vi "Double FFT Mesurament (Max Bin detection - Control - Init Wave&Window - Snapshot - DoubleFFT - Latency) RT Test.vi"() -> ()   [LabVIEW 2014]
uses:
  <vilib>/Platform/TimedLoop/XDataNode/timing_clust.ctl
  <vilib>/Platform/TimedLoop/XDataNode/nitl_modes.ctl
  <vilib>/Platform/TimedLoop/XDataNode/wakeup.ctl
  <vilib>/FPGAPlugInAG/sbRIO-9636/niLvFpga_Open_sbRIO-9636.vi
  <vilib>/rvi/interface/common/dynamic/niFpgaDynamicAddResources.vi
  <vilib>/Utility/error.llb/Error Cluster From Error Code.vi
  <vilib>/rvi/errors/niLvFpgaAdjustHostInterfaceError.vi
  <vilib>/rvi/interface/common/niFpgaWaitOnOcc.vi
  <vilib>/FPGAPlugInAG/Dynamic/niLvFpga_Run_Dynamic.vi
  <vilib>/FPGAPlugInAG/Dynamic/niLvFpga_Abort_Dynamic.vi
  <vilib>/FPGAPlugInAG/Dynamic/niLvFpga_Reset_Dynamic.vi
  <vilib>/FPGAPlugInAG/Dynamic/niLvFpga_Close_Dynamic.vi
  <vilib>/rvi/interface/nirviOpenFPGA/nirviOpenFPGA.xnode
  FPGA Bitfiles/LaserDistanceSen_FPGATarget_DoubleFFTMesuram_3rzWOSKuVyU.lvbitx
  FPGA Target/Test VIs/Double FFT Mesurament (Max Bin detection - Control - Init Wave&Window - Snapshot - DoubleFFT - Latency) test.vi
  <vilib>/rvi/interface/nirviReadWriteControl/nirviReadWriteControl.xnode
  <vilib>/rvi/interface/nirviMethod/nirviMethod.xnode
  <vilib>/Platform/TimedLoop/XDataNode/XDataNode.xnode
  <vilib>/rvi/interface/nirviCloseFPGA/nirviCloseFPGA.xnode
  <vilib>/FPGAPlugInAG/Dynamic/niLvFpga_ConfigureFifo_Dynamic.vi
  <vilib>/rvi/errors/niLvFpgaMergeErrorWithErrorCode.vi
  <vilib>/FPGAPlugInAG/Dynamic/niLvFpga_StartFifo_Dynamic.vi
  <vilib>/rvi/interface/Simulation/niFpgaSimulationCallBeginRW.vi
  <vilib>/FPGAPlugInAG/Dynamic/niLvFpga_ReadFifo_Dynamic.vi
  <vilib>/Platform/TimedLoop/XDataNode/XDNodeRunTimeDep.lvlib
  NiFpgaLv.dll
panel:
  in  "Initial Latency points":u32(slide)=50 scale=0.0..1249.0
  out "Second FFT (bin)":dbl[](graph)
  out "Second Signal (points) - Rising Triangular":dbl[](graph)
  out "Elements Remaining FFT":u32
  out "Elements Remaining Signal":u32
  out "First FFT (bin)":dbl[](graph)
  out "First Signal (points) - Falling Triangular":dbl[](graph)
  in  "Snapshot":bool
  in  "Windowing":T1(ring)
  in  "first bin":i32=10
  in  "last bin":i32=255
  in  "lower limit 2":u32(slide)=677 scale=625.0..738.0
  in  "lower limit 1":u32(slide)=59 scale=0.0..113.0
  out "Detected Frequency Tone - (Hz)":dbl
  in  "stop":bool
  out "Max Bin":i32
  out "Max Amp":dbl format="%.2f"
  out "Prev Bin":i32
  out "Next Bin":i32
  out "Prev Amp":dbl format="%.2f"
  out "Next Amp":dbl format="%.2f"
  out "Interpolated Bin":dbl
  in  "Interpolation Method":T2(ring)=enum."Jain"
  # "WARNING:\nOnce pressed wait untill the end of operation"
  # "ONLINE parameter"
  # "OFFLINE parameters"
  # "Max Detection FFT bin range"
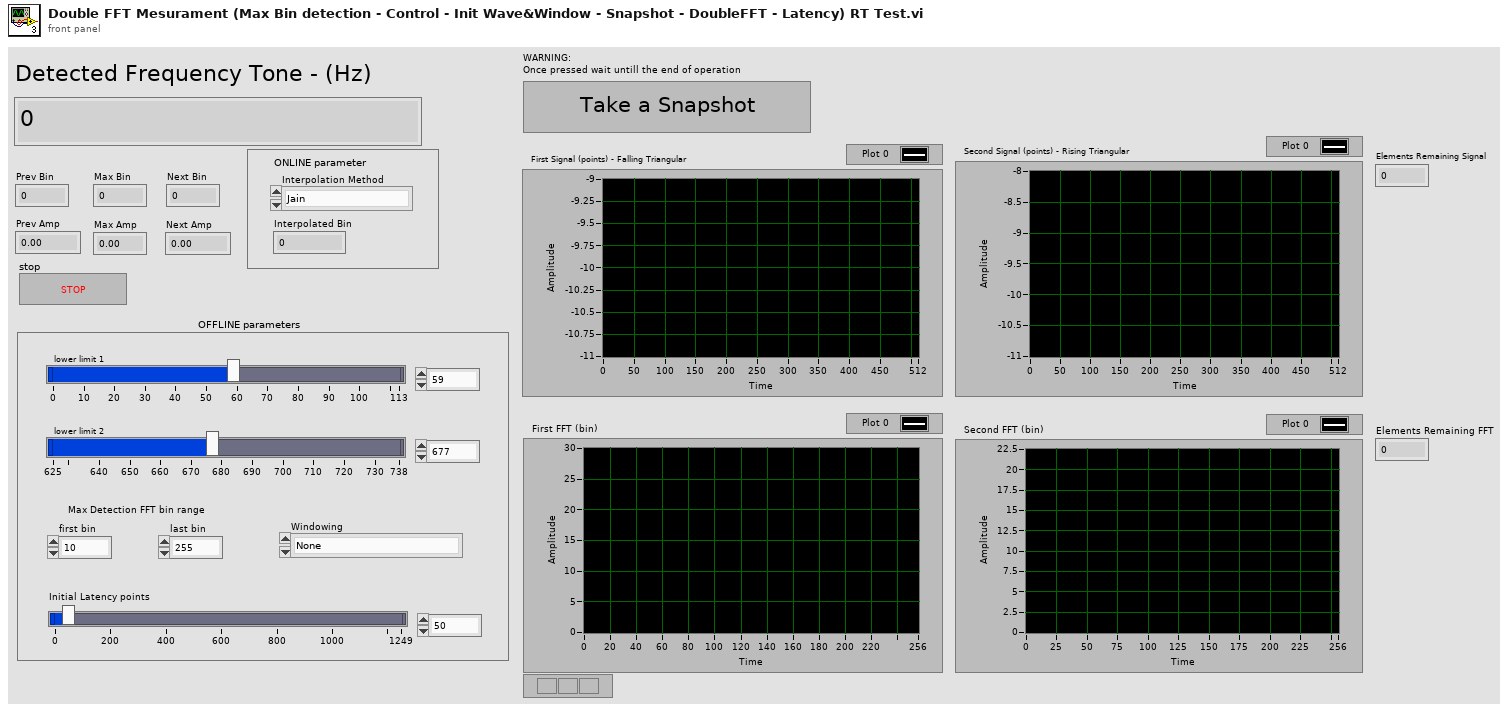
[diagram p1: front panel]
types:
  T1 = enum16{"None", "Hanning", "Hamming", "Blackman", "Blackman-Harris"}
  T2 = enum16{"Quadratic", "McLeodd", "Barycentric", "Jain"}
  T3 = typedef "XDNodeRunTimeDep.lvlib/timing_clust.ctl" = cluster{"Expected End [f-1]":u64, "Actual End [f-1]":u64, "Finished Late? [f-1]":bool, "Expected End [i-1]":u64, "Actual End [i-1]":u64, "Finished Late? [i-1]":bool, "Expected Start [i]":u64, "Actual Start [i]":u64, "Expected Start [f]":u64, "Actual Start [f]":u64, "Source Name":string, "Structure Name":string, "Period":i64, "Deadline":i64, "Offset":i64, "Start":i64, "Priority":i32, "Timeout":i32, "Mode":T4, "Wakeup Reason":T5, "Error":errorcluster, "Source Type":string, "Secondary Source Type":string, "Global End Time":u64, "Global Start Time":u64, "Frame Duration":u64, "Iteration Duration":u64, "Assigned CPU":i32, "I/O Scan Engine Mode":u32}
  T4 = typedef "XDNodeRunTimeDep.lvlib/nitl_modes.ctl" = enum32{"No Change", "Process missed periods, maintain original phase", "Discard missed periods, maintain original phase", "Process missed periods, ignore original phase", "Discard missed periods, ignore original phase"}
  T5 = typedef "XDNodeRunTimeDep.lvlib/wakeup.ctl" = enum32{"Normal", "Aborted", "Asynchronous wakeup", "Timing source error", "Timed loop error", "Timeout"}
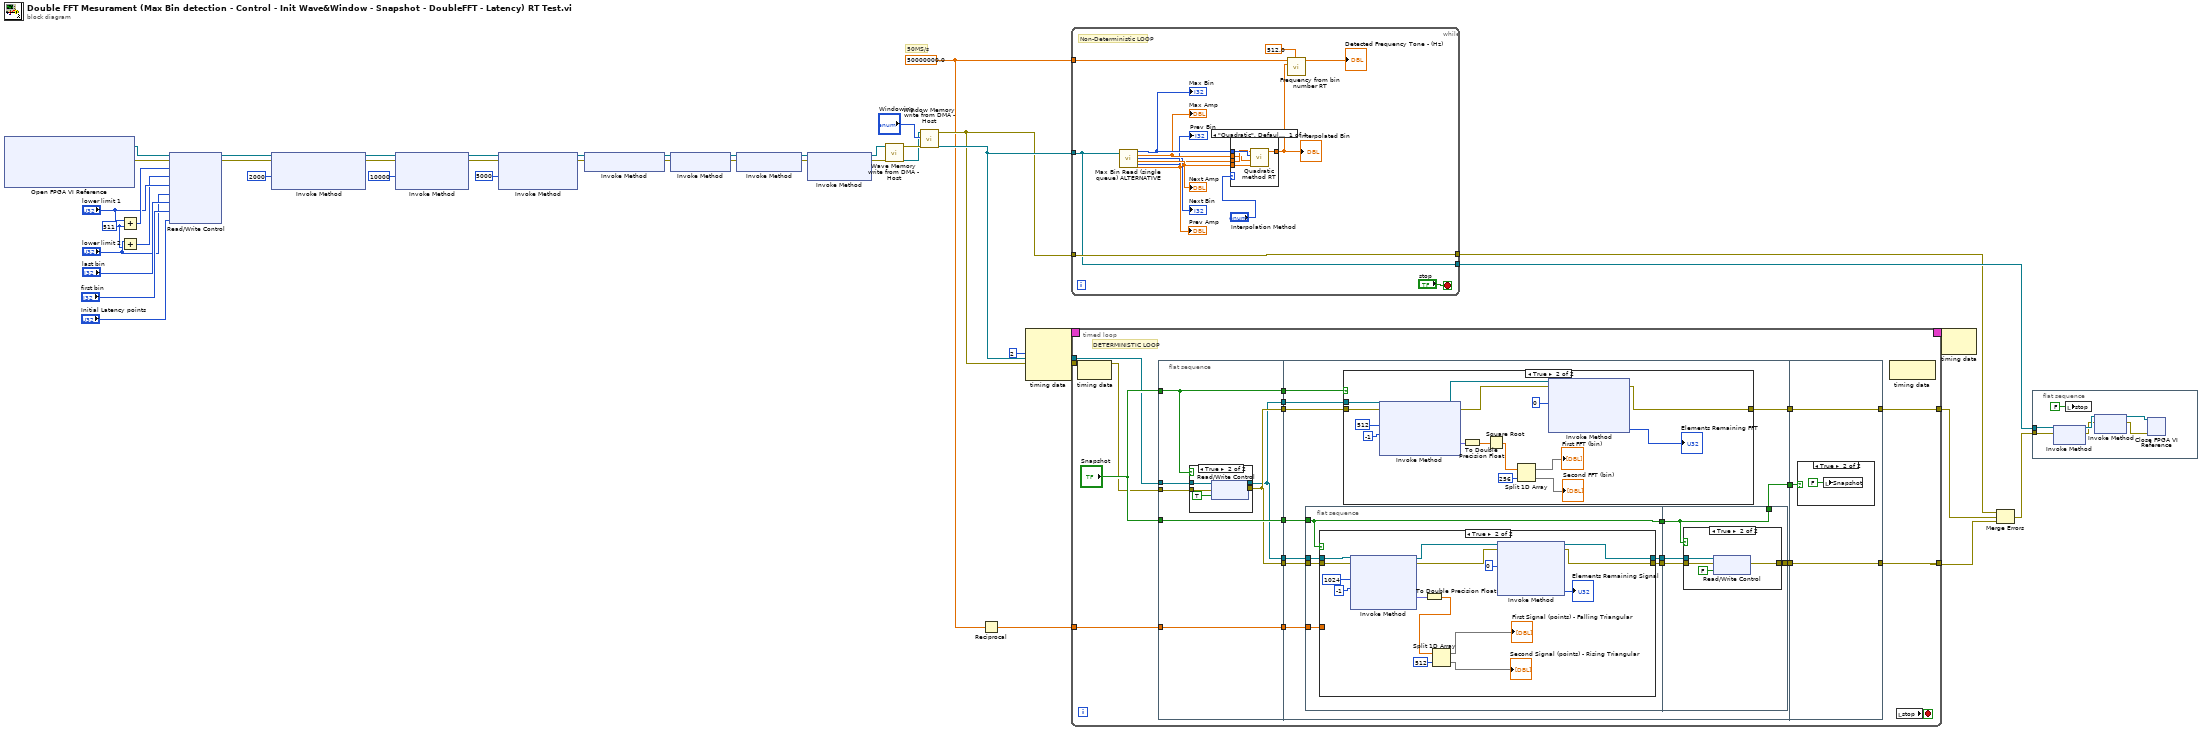
[diagram p0: block diagram]
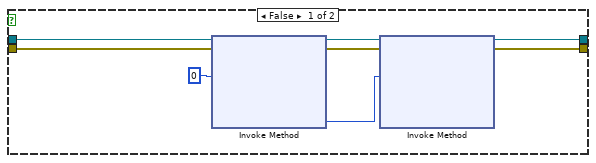
[diagram p3: hidden frame]
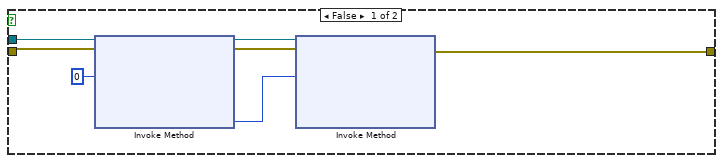
[diagram p5: hidden frame]
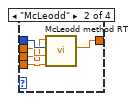
[diagram p7: hidden frame]
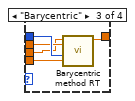
[diagram p8: hidden frame]
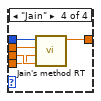
[diagram p9: hidden frame]
diagram:
  w38 = u32 511 ("y")
  w16 = 50000000.0 ("Sample Rate (S/s)")
  # "50MS/s"
  n1 = xnode "Open FPGA VI Reference"() -> ("FPGA VI Reference Out"=w37:refnum<k20>, "error out"=w36:errorcluster)  [unwired: 2 in]
  n2 = Add(x="lower limit 1", y=w38) -> (x+y=w42:u32)
  n3 = Add(x="lower limit 2", y=w38) -> (x+y=w40:u32)
  n4 = xnode "Read/Write Control"("FPGA VI Reference In"=w37, "error in"=w36, "upper limit 1"=w42, "upper limit 2"=w40, "lower limit 1"="lower limit 1", "lower limit 2"="lower limit 2", "last bin"="last bin", "first bin"="first bin", "Latency points"="Initial Latency points") -> ("FPGA VI Reference Out"=w31:refnum<k20>, "error out"=w30:errorcluster)
  n5 = xnode "Invoke Method"("FPGA VI Reference In"=w31, "error in"=w30, "Requested Depth"=u32 2000) -> ("FPGA VI Reference Out"=w29:refnum<k20>, "error out"=w28:errorcluster)  [unwired: 1 out]
  n6 = xnode "Invoke Method"("FPGA VI Reference In"=w29, "error in"=w28, "Requested Depth"=u32 10000) -> ("FPGA VI Reference Out"=w27:refnum<k20>, "error out"=w26:errorcluster)  [unwired: 1 out]
  n7 = xnode "Invoke Method"("FPGA VI Reference In"=w27, "error in"=w26, "Requested Depth"=u32 5000) -> ("FPGA VI Reference Out"=w10:refnum<k20>, "error out"=w11:errorcluster)  [unwired: 1 out]
  n8 = xnode "Invoke Method"("FPGA VI Reference In"=w10, "error in"=w11) -> ("FPGA VI Reference Out"=w20:refnum<k20>, "error out"=w19:errorcluster)
  n9 = xnode "Invoke Method"("FPGA VI Reference In"=w20, "error in"=w19) -> ("FPGA VI Reference Out"=w22:refnum<k20>, "error out"=w21:errorcluster)
  n10 = xnode "Invoke Method"("FPGA VI Reference In"=w22, "error in"=w21) -> ("FPGA VI Reference Out"=w8:refnum<k20>, "error out"=w9:errorcluster)
  n11 = xnode "Invoke Method"("FPGA VI Reference In"=w8, "error in"=w9) -> ("FPGA VI Reference Out"=w15:refnum<k20>, "error out"=w14:errorcluster)  [unwired: 1 in]
  n12 = call "Wave Memory write from DMA - Host.vi"("error in"=w14, "FPGA VI Reference In"=w15) -> ("FPGA VI Reference Out"=w12:refnum<k20>, "error out"=w13:errorcluster)  [unwired: 7 in, 1 out]
  n13 = call "Window Memory write from DMA - Host.vi"("error in"=w13, "Enum"="Windowing", "FPGA VI Reference In"=w12) -> ("FPGA VI Reference Out"=w33:refnum<k20>, "error out"=w32:errorcluster)  [unwired: 5 in, 2 out]
  n14 = Reciprocal(x=w16) -> (1/x=w17:dbl)
  n15 = node-c288(i64 2 ("Period")) -> (w7:T3)  [unwired: 3 in]
  n16 = while {
    tunnel: w16 -> [w57]
    tunnel: w33 -> [w55]
    tunnel: w32 -> [w56]
    tunnel: [w55] -> w35
    tunnel: [w56] -> w3
    stop <- "stop" stop-if-true
    # "Non-Deterministic LOOP"
    n17 = call "Max Bin Read (single queue) ALTERNATIVE.vi"("FPGA VI Reference In"=w55) -> ("Max Bin"=w51:i32, "Max Amp"=w50:dbl, "Next Bin"=→"Next Bin":i32, "Next Amp"=w49:dbl, "Prev Bin"=→"Prev Bin":i32, "Prev Amp"=w48:dbl)  [unwired: 12 in, 1 out]
    "Max Bin" <- w51
    "Max Amp" <- w50
    "Prev Amp" <- w48
    "Next Amp" <- w49
    n18 = case shown="\"Quadratic\", Default" "Interpolation Method" {
      tunnel: w51 -> [w62 w67 w72 w77]
      tunnel: w50 -> [w59 w66 w71 w76]
      tunnel: w48 -> [w60 w65 w70 w75]
      tunnel: w49 -> [w61 w64 w69 w74]
      tunnel: [w63 w68 w73 w78] -> w52
      frame "Quadratic", Default {
        n19 = call "Quadratic method RT.vi"("Next Amplitude"=w61, "Max Amplitude"=w59, "Max bin"=w62, "Prev Amplitude"=w60) -> ("Bin"=w63:dbl)  [unwired: 7 in]
      }
      frame "McLeodd" {
        n20 = call "McLeodd method RT.vi"("Next Amp"=w64, "Max Amp"=w66, "Max Bin"=w67, "Prev Amp"=w65) -> ("Bin"=w68:dbl)  [unwired: 7 in]
      }
      frame "Barycentric" {
        n21 = call "Barycentric method RT.vi"("Next Amp"=w69, "Max Bin"=w72, "Max Amp"=w71, "Prev Amp"=w70) -> ("Bin"=w73:dbl)  [unwired: 7 in]
      }
      frame "Jain" {
        n22 = call "Jain's method RT.vi"("Prev Amp"=w75, "Next Amp"=w74, "Max Amp"=w76, "Max Bin"=w77) -> ("Bin"=w78:dbl)  [unwired: 7 in]
      }
    }
    "Interpolated Bin" <- w52
    n23 = call "Frequency from bin number RT.vi"("FFT size"=512.0, "Bin number"=w52, "Sample Rate (S/s)"=w57) -> ("Detected Frequency (Hz)"=→"Detected Frequency Tone - (Hz)":dbl)  [unwired: 8 in]
  }
  n24 = timed-loop {
    tunnel: w33 -> [w89]
    tunnel: w32 -> [w90]
    tunnel: [w92] -> w4
    tunnel: w17 -> [w94]
    tunnel: [w93] -> w2
    timing: w7 -> [_]
    timing-out: [_] -> w6
    stop <- w95 stop-if-true
    # "DETERMINISTIC LOOP"
    n25 = node-c288() -> ()  [unwired: 1 in, 1 out]
    n26 = flat-sequence {
      tunnel: w89 -> [w100]
      tunnel: w90 -> [w101]
      tunnel: "Snapshot" -> [w98]
      tunnel: "Snapshot" -> [w103]
      tunnel: w94 -> [w104]
      tunnel: [w102] -> w88
      tunnel: [w104] -> w87
      tunnel: [w103] -> w86
      tunnel: [w98] -> w85
      tunnel: [w102] -> w84
      tunnel: [w99] -> w83
      tunnel: [w99] -> w82
      tunnel: w88 -> [w120]
      tunnel: w87 -> [w119]
      tunnel: w86 -> [w113]
      tunnel: w85 -> [w116]
      tunnel: w84 -> [w115]
      tunnel: w83 -> [w114]
      tunnel: w82 -> [w121]
      tunnel: [w118] -> w81
      tunnel: [w117] -> w80
      tunnel: [w112] -> w79
      tunnel: [w186] -> w92
      tunnel: [w187] -> w93
      tunnel: w81 -> [w187]
      tunnel: w80 -> [w186]
      tunnel: w79 -> [w185]
      frame #0 {
        n27 = case shown="True" w98 {
          tunnel: [w105 w110] -> w102
          tunnel: w101 -> [w105 w109]
          tunnel: w100 -> [w106 w108]
          tunnel: [w106 w107] -> w99
          frame False {
          }
          frame True {
            n28 = xnode "Read/Write Control"("FPGA VI Reference In"=w108, "error in"=w109, "snapshot"=TRUE) -> ("FPGA VI Reference Out"=w107:refnum<k20>, "error out"=w110:errorcluster)
          }
        }
      }
      frame #1 {
        n29 = flat-sequence {
          tunnel: w121 -> [w130]
          tunnel: w120 -> [w129]
          tunnel: w119 -> [w128]
          tunnel: w113 -> [w125]
          tunnel: [w127] -> w124
          tunnel: [w126] -> w123
          tunnel: [w125] -> w122
          tunnel: [w155] -> w117
          tunnel: w124 -> [w157]
          tunnel: w123 -> [w156]
          tunnel: w122 -> [w154]
          tunnel: [w154] -> w112
          frame #0 {
            n30 = case shown="True" w125 {
              tunnel: w130 -> [w137 w153]
              tunnel: w129 -> [w135 w152]
              tunnel: [w134 w145] -> w126
              tunnel: w128 -> [_ _]
              tunnel: [w131 w144] -> w127
              frame False {
                n31 = xnode "Invoke Method"("FPGA VI Reference In"=w137, "error in"=w135, "Number of Elements"=u32 0) -> ("FPGA VI Reference Out"=w133:refnum<k20>, "error out"=w132:errorcluster, "Elements Remaining"=w136:u32)  [unwired: 1 in, 1 out]
                n32 = xnode "Invoke Method"("FPGA VI Reference In"=w133, "error in"=w132, "Number of Elements"=w136) -> ("FPGA VI Reference Out"=w131:refnum<k20>, "error out"=w134:errorcluster)  [unwired: 1 in, 2 out]
              }
              frame True {
                n33 = xnode "Invoke Method"("FPGA VI Reference In"=w153, "error in"=w152, "Number of Elements"=u32 1024, "Timeout (ms)"=-1) -> ("FPGA VI Reference Out"=w147:refnum<k20>, "error out"=w146:errorcluster, "Data"=w149:fxp<+/-,12,12>[])  [unwired: 1 out]
                n34 = To Double Precision Float(number=w149) -> (double precision float=w142:dbl[])
                n35 = Split 1D Array(array=w142, index=512) -> (first subarray=→"First Signal (points) - Falling Triangular":dbl[], second subarray=→"Second Signal (points) - Rising Triangular":dbl[])
                n36 = xnode "Invoke Method"("FPGA VI Reference In"=w147, "error in"=w146, "Number of Elements"=u32 0) -> ("FPGA VI Reference Out"=w144:refnum<k20>, "error out"=w145:errorcluster, "Elements Remaining"=→"Elements Remaining Signal":u32)  [unwired: 1 in, 1 out]
              }
            }
          }
          frame #1 {
            n37 = case shown="True" w154 {
              tunnel: [w158 w160] -> w155
              tunnel: w157 -> [_ w161]
              tunnel: w156 -> [w158 w159]
              frame False {
              }
              frame True {
                n38 = xnode "Read/Write Control"("FPGA VI Reference In"=w161, "error in"=w159, "snapshot"=FALSE) -> ("error out"=w160:errorcluster)  [unwired: 1 out]
              }
            }
          }
        }
        n39 = case shown="True" w116 {
          tunnel: w114 -> [w168 w179]
          tunnel: w115 -> [w165 w180]
          tunnel: [w164 w178] -> w118
          frame False {
            n40 = xnode "Invoke Method"("FPGA VI Reference In"=w168, "error in"=w165, "Number of Elements"=u32 0) -> ("FPGA VI Reference Out"=w166:refnum<k20>, "error out"=w163:errorcluster, "Elements Remaining"=w167:u32)  [unwired: 1 in, 1 out]
            n41 = xnode "Invoke Method"("FPGA VI Reference In"=w166, "error in"=w163, "Number of Elements"=w167) -> ("error out"=w164:errorcluster)  [unwired: 1 in, 3 out]
          }
          frame True {
            n42 = xnode "Invoke Method"("FPGA VI Reference In"=w179, "error in"=w180, "Number of Elements"=u32 512, "Timeout (ms)"=-1) -> ("FPGA VI Reference Out"=w176:refnum<k20>, "error out"=w177:errorcluster, "Data"=w182:fxp<+,44,44>[])  [unwired: 1 out]
            n43 = To Double Precision Float(number=w182) -> (double precision float=w181:dbl[])
            n44 = Square Root(x=w181) -> (sqrt(x)=w171:dbl[])
            n45 = Split 1D Array(array=w171, index=256) -> (first subarray=→"First FFT (bin)":dbl[], second subarray=→"Second FFT (bin)":dbl[])
            n46 = xnode "Invoke Method"("FPGA VI Reference In"=w176, "error in"=w177, "Number of Elements"=u32 0) -> ("error out"=w178:errorcluster, "Elements Remaining"=→"Elements Remaining FFT":u32)  [unwired: 1 in, 2 out]
          }
        }
      }
      frame #2 {
        n47 = case shown="True" w185 {
          frame False {
          }
          frame True {
            n48 = local write "Snapshot"(FALSE ("Snapshot")) -> ()
          }
        }
      }
    }
    n49 = node-c288() -> ()  [unwired: 1 in, 1 out]
    n50 = local read "stop"() -> (w95:bool)
  }
  n51 = node-c288(w6) -> ()  [unwired: 1 out]
  n52 = Merge Errors(w3, w2, w4) -> (w18:errorcluster)
  n53 = flat-sequence {
    tunnel: w35 -> [w195]
    tunnel: w18 -> [w194]
    frame #0 {
      n54 = xnode "Invoke Method"("FPGA VI Reference In"=w195, "error in"=w194) -> ("FPGA VI Reference Out"=w190:refnum<k20>, "error out"=w189:errorcluster)
      n55 = local write "stop"(FALSE ("stop")) -> ()
      n56 = xnode "Invoke Method"("FPGA VI Reference In"=w190, "error in"=w189) -> ("FPGA VI Reference Out"=w191:refnum<k20>, "error out"=w192:errorcluster)
      n57 = xnode "Close FPGA VI Reference"("FPGA VI Reference In"=w191, "error in"=w192) -> ()  [unwired: 1 out]
    }
  }
